vi "Open Reentrant VI.vi"(8 "error in (no error)":errorcluster, 10 "Message":T1={"Source"="", "Destination"="", "Time Stamp"=timestamp(0 s since 1904-01-01), "Command"="", "Data"=variant(string "")}, 11 "VI Path":path) -> (0 "error out":errorcluster, 1 "Clone Name":string, 2 "VI Refnum":refnum<vi>, 3 "queue out":refnum<queue>)   [LabVIEW 2018]
doc: "Opens the VI at the specified path in Reentrant Mode (0x08). If a command was specified in the initial message, the initial message is sent to the new reentrant VI. The correct destination field for the initial message will be set by this VI."
uses:
  <userlib>/Dynamic Reentrant/Type Defs/Message.ctl
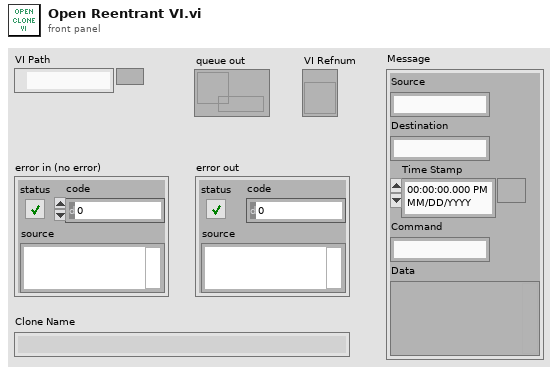
[diagram p1: front panel]
types:
  T1 = typedef "Message.ctl" = cluster{"Source":string, "Destination":string, "Time Stamp":timestamp, "Command":string, "Data":variant}
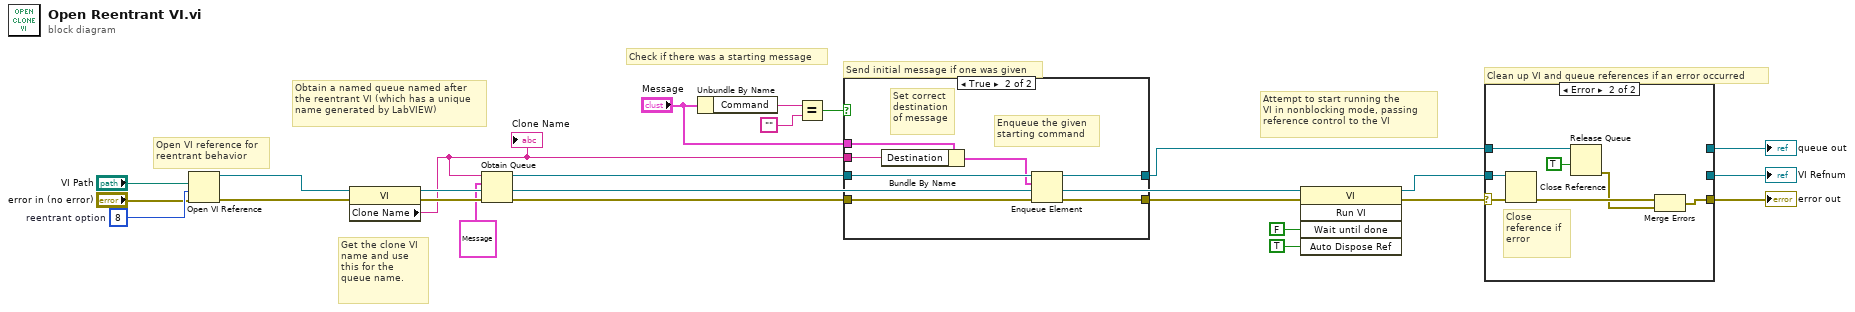
[diagram p0: block diagram]
diagram:
  w16 = 8  # reentrant option
  # "Clean up VI and queue references if an error occurred"
  # "Send initial message if one was given"
  # "Check if there was a starting message"
  # "Get the clone VI name and use this for the queue name."
  # "Attempt to start running the\nVI in nonblocking mode, passing\nreference control to the VI"
  # "Obtain a named queue named after\nthe reentrant VI (which has a unique\nname generated by LabVIEW)"
  # "Open VI reference for\nreentrant behavior"
  n1 = Open VI Reference(vi path="VI Path", options=w16, error in (no error)="error in (no error)") -> (vi reference=w22:refnum<vi>, error out=w21:errorcluster)  [unwired: 3 in]
  n2 = property class="VI"(reference=w22, error in=w21) -> (reference out=w15:refnum<vi>, error out=w19:errorcluster, "Clone Name"=w8:string)
  "Clone Name" <- w8
  n3 = Obtain Queue(name (unnamed)=w8, element data type=T1 {"Source"="", "Destination"="", "Time Stamp"=timestamp(0 s since 1904-01-01), "Command"="", "Data"=variant(string "")} ("Message"), error in (no error)=w19) -> (queue out=w7:refnum<queue>, error out=w13:errorcluster)  [unwired: 2 in, 1 out]
  n4 = Unbundle By Name("Message") -> ("Command"=w6:string)
  n5 = Equal?(x=w6, y="") -> (x = y?=w4:bool)
  n6 = case shown="True" w4 {
    tunnel: [w25 w33] -> w23
    tunnel: w13 -> [w25 w32]
    tunnel: w8 -> [_ w31]
    tunnel: w7 -> [w26 w30]
    tunnel: [w26 w29] -> w2
    tunnel: "Message" -> [_ w27]
    frame False {
    }
    frame True {
      # "Set correct \ndestination\nof message"
      # "Enqueue the given \nstarting command"
      n7 = Bundle By Name(cluster=w27, "Destination"=w31) -> (w28:T1)
      n8 = Enqueue Element(queue=w30, element=w28, error in (no error)=w32) -> (queue out=w29:refnum<queue>, error out=w33:errorcluster)  [unwired: 1 in, 1 out]
    }
  }
  n9 = invoke class="VI" method="Run VI"(reference=w15, error in=w23, "Wait until done"=FALSE, "Auto Dispose Ref"=TRUE) -> (reference out=w14:refnum<vi>, error out=w24:errorcluster)  [unwired: 1 in, 3 out]
  n10 = case shown="Error" w24 {
    selector: w24 -> [w36 w43]
    tunnel: w14 -> [w35 w42]
    tunnel: [w36 w38] -> w11
    tunnel: [w35 _] -> w10
    tunnel: w2 -> [w34 w40]
    tunnel: [w34 _] -> w1
    frame No Error {
    }
    frame Error {
      # "Close reference if error"
      n11 = Close Reference(reference=w42, error in (no error)=w43) -> (error out=w41:errorcluster)
      n12 = Release Queue(queue=w40, force destroy? (F)=TRUE) -> (error out=w37:errorcluster)  [unwired: 1 in, 2 out]
      n13 = Merge Errors(w41, w37) -> (w38:errorcluster)
    }
  }
  "error out" <- w11
  "VI Refnum" <- w10
  "queue out" <- w1
